vi "SwerveDrive.vi"   [LabVIEW 2019]
doc: "This VI runs in parallel to other tasks. It can contain as many user-defined periodic loops as you need. These can carry out PID or other sorts of timed response."
uses:
  <vilib>/Rock Robotics/WPI/ThirdParty/Phoenix-LabVIEW/Motor Controller/Controls/CTRE_Phoenix_MotorControl_ControlMode.ctl
  <vilib>/Rock Robotics/WPI/Utilities/WPI_GetSetVariantRefNum.vi
  <vilib>/Rock Robotics/Network Tables/NT Read Numeric Array.vi
  <vilib>/Rock Robotics/Network Tables/NT Write Numeric Array.vi
  Program Files/navX.Library.v2/navX Library v2/navX Library v2.lvlib
types:
  T1 = typedef "WPI_AnalogChannelDevRef.ctl" = cluster{"DevStatus":errorcluster, "Analog Channel":T2}
  T2 = typedef "FPGA_AIChannel.ctl" = enum8{"AI 0", "AI 1", "AI 2", "AI 3", "AI MXP 0", "AI MXP 1", "AI MXP 2", "AI MXP 3", "Invalid"}
  T3 = typedef "WPI_JoystickDevRef.ctl" = cluster{"Device":T4}
  T4 = typedef "WPI_JoystickDeviceEnum.ctl" = enum16{"USB 0", "USB 1", "USB 2", "USB 3", "USB 4", "USB 5"}
  T5 = typedef "WPI_MotorControlDeviceRef.ctl" = cluster{"DeviceStatus":errorcluster, "Type":T6, "PWM":cluster{"PWM Channel":T7, "DeadBand":T8}, "CAN":cluster{"Device Number":u8, "SetOutput VI Ref":variant, "GetOutput VI Ref":variant, "Enable VI Ref":variant, "Disable VI Ref":variant, "Data":variant}, "Invert":bool, "DIO PWM":cluster{"PWM \"Enable\" Channel":T7, "DIOChannel":T9, "PWM Rate":dbl}}
  T6 = typedef "WPI_MotorControlType.ctl" = enum16{"PWM", "CAN", "DIO PWM"}
  T7 = typedef "FPGA_DIOPWMChannel.ctl" = enum8{"PWM 0", "PWM 1", "PWM 2", "PWM 3", "PWM 4", "PWM 5", "PWM 6", "PWM 7", "PWM 8", "PWM 9", "PWM MXP 0", "PWM MXP 1", "PWM MXP 2", "PWM MXP 3", "PWM MXP 4", "PWM MXP 5", "PWM MXP 6", "PWM MXP 7", "PWM MXP 8", "PWM MXP 9", "Invalid"}
  T8 = typedef "WPI_PWMDeadband.ctl" = cluster{"Name":string, "maxPositivePwm":i32, "minPositivePwm":i32, "centerPwm":i32, "maxNegativePwm":i32, "minNegativePwm":i32, "angularRange":u16}
  T9 = typedef "FPGA_DIOChannel.ctl" = enum8{"DIO 0", "DIO 1", "DIO 2", "DIO 3", "DIO 4", "DIO 5", "DIO 6", "DIO 7", "DIO 8", "DIO 9", "DIO MXP 0", "DIO MXP 1", "DIO MXP 2", "DIO MXP 3", "DIO MXP 4", "DIO MXP 5", "DIO MXP 6", "DIO MXP 7", "DIO MXP 8", "DIO MXP 9", "DIO MXP 10", "DIO MXP 11", "DIO MXP 12", "DIO MXP 13", "DIO MXP 14", "DIO MXP 15", "SPI Port CS1", "SPI Port CS2", "SPI Port CS3", "SPI Port MISO", "SPI Port MOSI", "Invalid"}
  T10 = cluster{"PhoenixMotorControlDevRef":T5, "PhoenixMotorControlDevRef":T5, "PhoenixMotorControlDevRef":T5, "PhoenixMotorControlDevRef":T5}
  T11 = typedef "CTRE_Phoenix_MotorControl_ControlMode.ctl" = u16
  T12 = typedef "navX Library v2.lvlib/Z900_navX_DeviceTypeDef.ctl" = cluster{"Interface":cluster{"Protocol":T13, "Update Rate (4Hz-100Hz)":u8, "navX Open TypeDef":variant}, "Notify Packet":refnum<notifier>, "Loop VI Refnum":refnum<vi>, "Ready to Close Occurrence Refnum":refnum<k4>}
  T13 = typedef "navX Library v2.lvlib/Z900_navX_ProtocolTypeDef.ctl" = enum16{"SERIAL", "I2C", "SPI"}
  T14 = cluster{"Yaw":dbl, "Roll":dbl, "Pitch":dbl, "Heading":dbl, "Fused Heading":dbl}
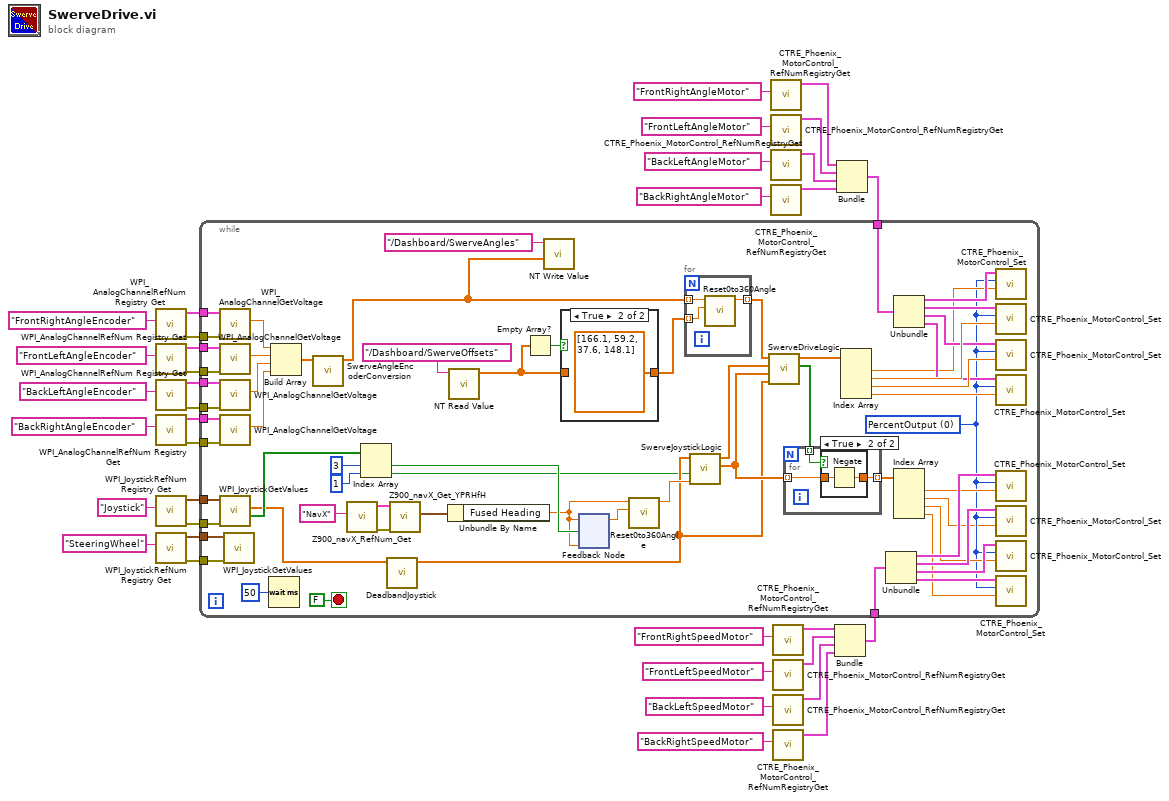
[diagram p0: block diagram]
diagram:
  n1 = call <vilib>:"WPI_AnalogChannelRefNum Registry Get.vi"("refnum name"="FrontRightAngleEncoder") -> ("error out"=w12:errorcluster, "AIDeviceRef"=w22:T1)  [unwired: 9 in]
  n2 = call <vilib>:"WPI_AnalogChannelRefNum Registry Get.vi"("refnum name"="FrontLeftAngleEncoder") -> ("error out"=w11:errorcluster, "AIDeviceRef"=w21:T1)  [unwired: 9 in]
  n3 = call <vilib>:"WPI_AnalogChannelRefNum Registry Get.vi"("refnum name"="BackLeftAngleEncoder") -> ("error out"=w10:errorcluster, "AIDeviceRef"=w20:T1)  [unwired: 9 in]
  n4 = call <vilib>:"WPI_AnalogChannelRefNum Registry Get.vi"("refnum name"="BackRightAngleEncoder") -> ("error out"=w9:errorcluster, "AIDeviceRef"=w19:T1)  [unwired: 9 in]
  n5 = call <vilib>:"WPI_JoystickRefNum Registry Get.vi"("refnum name"="Joystick") -> ("error out"=w6:errorcluster, "JoystickDevRef"=w7:T3)  [unwired: 1 in, 8 out]
  n6 = call <vilib>:"WPI_JoystickRefNum Registry Get.vi"("refnum name"="SteeringWheel") -> ("error out"=w4:errorcluster, "JoystickDevRef"=w5:T3)  [unwired: 1 in, 8 out]
  n7 = call <vilib>:"CTRE_Phoenix_MotorControl_RefNumRegistryGet.vi"("refnum name"="FrontRightAngleMotor") -> ("PhoenixMotorControlDevRef"=w13:T5)  [unwired: 9 in, 1 out]
  n8 = call <vilib>:"CTRE_Phoenix_MotorControl_RefNumRegistryGet.vi"("refnum name"="FrontLeftAngleMotor") -> ("PhoenixMotorControlDevRef"=w17:T5)  [unwired: 9 in, 1 out]
  n9 = call <vilib>:"CTRE_Phoenix_MotorControl_RefNumRegistryGet.vi"("refnum name"="BackLeftAngleMotor") -> ("PhoenixMotorControlDevRef"=w18:T5)  [unwired: 9 in, 1 out]
  n10 = call <vilib>:"CTRE_Phoenix_MotorControl_RefNumRegistryGet.vi"("refnum name"="BackRightAngleMotor") -> ("PhoenixMotorControlDevRef"=w15:T5)  [unwired: 9 in, 1 out]
  n11 = call <vilib>:"CTRE_Phoenix_MotorControl_RefNumRegistryGet.vi"("refnum name"="FrontRightSpeedMotor") -> ("PhoenixMotorControlDevRef"=w16:T5)  [unwired: 9 in, 1 out]
  n12 = call <vilib>:"CTRE_Phoenix_MotorControl_RefNumRegistryGet.vi"("refnum name"="FrontLeftSpeedMotor") -> ("PhoenixMotorControlDevRef"=w3:T5)  [unwired: 9 in, 1 out]
  n13 = call <vilib>:"CTRE_Phoenix_MotorControl_RefNumRegistryGet.vi"("refnum name"="BackLeftSpeedMotor") -> ("PhoenixMotorControlDevRef"=w23:T5)  [unwired: 9 in, 1 out]
  n14 = call <vilib>:"CTRE_Phoenix_MotorControl_RefNumRegistryGet.vi"("refnum name"="BackRightSpeedMotor") -> ("PhoenixMotorControlDevRef"=w24:T5)  [unwired: 9 in, 1 out]
  n15 = Bundle("PhoenixMotorControlDevRef"=w16, "PhoenixMotorControlDevRef"=w3, "PhoenixMotorControlDevRef"=w23, "PhoenixMotorControlDevRef"=w24) -> (w8:T10)  [unwired: 1 in]
  n16 = Bundle("PhoenixMotorControlDevRef"=w13, "PhoenixMotorControlDevRef"=w17, "PhoenixMotorControlDevRef"=w18, "PhoenixMotorControlDevRef"=w15) -> (w14:T10)  [unwired: 1 in]
  n17 = while {
    tunnel: w22 -> [w75]
    tunnel: w21 -> [w70]
    tunnel: w20 -> [w67]
    tunnel: w19 -> [w73]
    tunnel: w14 -> [w83]
    tunnel: w12 -> [w76]
    tunnel: w11 -> [w69]
    tunnel: w10 -> [w66]
    tunnel: w9 -> [w72]
    tunnel: w8 -> [w61]
    tunnel: w7 -> [w57]
    tunnel: w6 -> [w56]
    tunnel: w5 -> [w55]
    tunnel: w4 -> [w54]
    stop <- FALSE stop-if-true
    w77 = T11 0 items=["PercentOutput"=0, "Position"=1, "Velocity"=2, "Current"=3, "Follower"=5, "MotionProfile"=6, "MotionMagic"=7, "MotionProfileArc"=10, "Disabled"=15] ("Control Mode")
    n18 = call <vilib>:"WPI_AnalogChannelGetVoltage.vi"("error in (no error)"=w76, "AIDeviceRef"=w75) -> ("Voltage"=w74:dbl)  [unwired: 7 in, 2 out]
    n19 = call <vilib>:"WPI_AnalogChannelGetVoltage.vi"("error in (no error)"=w69, "AIDeviceRef"=w70) -> ("Voltage"=w68:dbl)  [unwired: 7 in, 2 out]
    n20 = call <vilib>:"WPI_AnalogChannelGetVoltage.vi"("error in (no error)"=w66, "AIDeviceRef"=w67) -> ("Voltage"=w65:dbl)  [unwired: 7 in, 2 out]
    n21 = call <vilib>:"WPI_AnalogChannelGetVoltage.vi"("error in (no error)"=w72, "AIDeviceRef"=w73) -> ("Voltage"=w71:dbl)  [unwired: 7 in, 2 out]
    n22 = call <vilib>:"WPI_JoystickGetValues.vi"("error in (no error)"=w56, "JoystickDevRef"=w57) -> ("Buttons"=w60:bool[], "Axes"=w38:dbl[])  [unwired: 5 in, 3 out]
    n23 = call <vilib>:"WPI_JoystickGetValues.vi"("error in (no error)"=w54, "JoystickDevRef"=w55) -> ()  [unwired: 5 in, 5 out]
    n24 = Wait (ms)(milliseconds to wait=u32 50) -> ()  [unwired: 1 out]
    n25 = Build Array(w74, w68, w65, w71) -> (w82:dbl[])
    n26 = call "SwerveAngleEncoderConversion.vi"("Voltages"=w82) -> ("Angles"=w48:dbl[])  [unwired: 10 in]
    n27 = call "Z900_navX_RefNum_Get.vi"("refnum name"="NavX") -> ("error out"=w44:errorcluster, "navX Device"=w45:T12)  [unwired: 9 in]
    n28 = Index Array(array=w60, index #1=3 ("index"), index #2=1 ("index")) -> (element #1=w41:bool, element #2=w39:bool)
    n29 = call "DeadbandJoystick.vi"("InputArray"=w38) -> ("OutputArray"=w40:dbl[])  [unwired: 10 in]
    n30 = call "Z900_navX_Get_YPRHfH.vi"("error in (no error)"=w44, "navX Device"=w45) -> ("YRPHfH"=w62:T14)  [unwired: 6 in, 3 out]
    n31 = Unbundle By Name(w62) -> ("Fused Heading"=w37:dbl)
    n32 = call-poly <vilib>:"NT Read Value.vi"("Name"="/Dashboard/SwerveOffsets") -> ("Numeric Array"=w53:dbl[])  [unwired: 9 in, 1 out]
    n33 = Empty Array?(array=w53) -> (empty?=w52:bool)
    n34 = call-poly <vilib>:"NT Write Value.vi"("Numeric Array"=w48, "Name"="/Dashboard/SwerveAngles") -> ()  [unwired: 9 in, 1 out]
    n35 = case shown="True" w52 {
      tunnel: [w101 dbl[] [166.1, 59.2, 37.6, 148.1] ("Numeric Array")] -> w51
      tunnel: w53 -> [w101 _]
      frame False {
      }
      frame True {
      }
    }
    n36 = feedback-in #1(w37, w41) -> ()
    n37 = feedback #1(w37) -> (w43:dbl)
    n38 = call "Reset0to360Angle.vi"("Offset"=w43, "AngleInput"=w37) -> ("AngleOutput"=w42:dbl)  [unwired: 9 in]
    n39 = for {
      tunnel: w48 -> [w104] mode=indexing
      tunnel: [w105] -> w88 mode=indexing
      tunnel: w51 -> [w103] mode=indexing
      n40 = call "Reset0to360Angle.vi"("Offset"=w103, "AngleInput"=w104) -> ("AngleOutput"=w105:dbl)  [unwired: 9 in]
    }
    n41 = call "SwerveJoystickLogic.vi"("Gyro"=w42, "TankMode"=w39, "Joystick Axes"=w40) -> ("Speeds"=w46:dbl[], "Angles"=w87:dbl[])  [unwired: 6 in]
    n42 = call "SwerveDriveLogic.vi"("Joystick Axes"=w40, "Speeds"=w46, "AngleSetpoints"=w87, "AngleEncoders"=w88) -> ("AngleMotorsReversed"=w89:bool[], "AngleMotorOutputs"=w86:dbl[])  [unwired: 6 in]
    n43 = for {
      tunnel: w46 -> [w107] mode=indexing
      tunnel: [w108] -> w94 mode=indexing
      tunnel: w89 -> [w106] mode=indexing
      n44 = case shown="True" w106 {
        tunnel: w107 -> [w109 w111]
        tunnel: [w109 w110] -> w108
        frame False {
        }
        frame True {
          n45 = Negate(x=w111) -> (-x=w110:dbl)
        }
      }
    }
    n46 = Index Array(array=w86) -> (element #1=w80:dbl, element #2=w99:dbl, element #3=w98:dbl, element #4=w81:dbl)  [unwired: 4 in]
    n47 = Unbundle(w61) -> ("PhoenixMotorControlDevRef"=w85:T5, "PhoenixMotorControlDevRef"=w93:T5, "PhoenixMotorControlDevRef"=w92:T5, "PhoenixMotorControlDevRef"=w91:T5)
    n48 = Unbundle(w83) -> ("PhoenixMotorControlDevRef"=w97:T5, "PhoenixMotorControlDevRef"=w96:T5, "PhoenixMotorControlDevRef"=w95:T5, "PhoenixMotorControlDevRef"=w90:T5)
    n49 = Index Array(array=w94) -> (element #1=w79:dbl, element #2=w63:dbl, element #3=w78:dbl, element #4=w64:dbl)  [unwired: 4 in]
    n50 = call <vilib>:"CTRE_Phoenix_MotorControl_Set.vi"("Output"=w80, "Control Mode"=w77, "PhoenixMotorControlDevRef"=w97) -> ()  [unwired: 7 in, 2 out]
    n51 = call <vilib>:"CTRE_Phoenix_MotorControl_Set.vi"("Output"=w99, "Control Mode"=w77, "PhoenixMotorControlDevRef"=w96) -> ()  [unwired: 7 in, 2 out]
    n52 = call <vilib>:"CTRE_Phoenix_MotorControl_Set.vi"("Output"=w98, "Control Mode"=w77, "PhoenixMotorControlDevRef"=w95) -> ()  [unwired: 7 in, 2 out]
    n53 = call <vilib>:"CTRE_Phoenix_MotorControl_Set.vi"("Output"=w81, "Control Mode"=w77, "PhoenixMotorControlDevRef"=w90) -> ()  [unwired: 7 in, 2 out]
    n54 = call <vilib>:"CTRE_Phoenix_MotorControl_Set.vi"("Output"=w79, "Control Mode"=w77, "PhoenixMotorControlDevRef"=w85) -> ()  [unwired: 7 in, 2 out]
    n55 = call <vilib>:"CTRE_Phoenix_MotorControl_Set.vi"("Output"=w63, "Control Mode"=w77, "PhoenixMotorControlDevRef"=w93) -> ()  [unwired: 7 in, 2 out]
    n56 = call <vilib>:"CTRE_Phoenix_MotorControl_Set.vi"("Output"=w78, "Control Mode"=w77, "PhoenixMotorControlDevRef"=w92) -> ()  [unwired: 7 in, 2 out]
    n57 = call <vilib>:"CTRE_Phoenix_MotorControl_Set.vi"("Output"=w64, "Control Mode"=w77, "PhoenixMotorControlDevRef"=w91) -> ()  [unwired: 7 in, 2 out]
  }
